vi "SelectionChangedRegEvent.vi"(0 "reference in":refnum<class "DataGridView.lvclass">, 11 "error in (no error)":errorcluster) -> (4 "reference out":refnum<class "DataGridView.lvclass">, 15 "error out":errorcluster)   [LabVIEW 2018, in "DataGridView.lvclass"]
uses:
  DataGridView.lvclass
  System.Windows.Forms
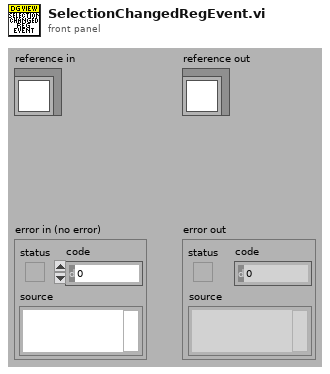
[diagram p1: front panel]
types:
  T1 = typedef "DataGridView.lvclass/ObjectAttributes.ctl" = cluster{"DataGridView":refnum<k24>, "SelectionChangedEvent":refnum<user-event>, "SelectionChanged callback ref":refnum<k27>, "LastSelectedRowIndex":i32, "CellClickEvent":refnum<user-event>, "CellClick callback refnum":refnum<k27>}
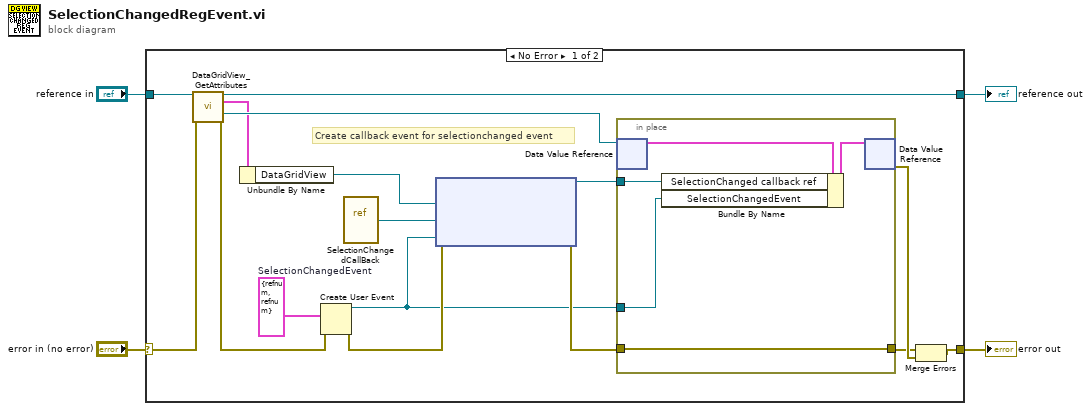
[diagram p0: block diagram]
diagram:
  n1 = case shown="No Error" "error in (no error)" {
    selector: "error in (no error)" -> [w16 w27]
    tunnel: [w14 w27] -> w3
    tunnel: [w18 w26] -> w1
    tunnel: "reference in" -> [w19 w26]
    frame No Error {
      w10 = cluster{"sender":refnum<k24>, "e":refnum<k24>} {"sender"=refnum, "e"=refnum}  # SelectionChangedEvent
      # "Create callback event for selectionchanged event"
      n2 = call "DataGridView_GetAttributes.vi"("reference in"=w19, "error in (no error)"=w16) -> ("reference out"=w18:refnum<class "DataGridView.lvclass">, "Data"=w11:T1, "DataRef"=w17:refnum<data-value>, "error out"=w7:errorcluster)  [unwired: 10 in]
      n3 = Unbundle By Name(w11) -> ("DataGridView"=w9:refnum<k24>)
      n4 = Create User Event(user event datatype=w10, error in=w7) -> (user event=w5:refnum<user-event>, error out=w6:errorcluster)
      n5 = vi-ref "SelectionChangedCallBack.vi"() -> ("vi reference"=w12:refnum<vi>)
      n6 = node(w6, w9, w12, w5) -> (w13:refnum<k27>, w8:errorcluster)  [unwired: 1 in]
      n7 = in-place {
        in-place-border: w8 -> [w24]
        in-place-border: [w24] -> w15
        in-place-border: w13 -> [w22]
        in-place-border: w5 -> [w21]
        n8 = in-place-dvr #1(w17) -> (w23:T1)  [unwired: 1 out]
        n9 = Bundle By Name(cluster=w23, "SelectionChanged callback ref"=w22, "SelectionChangedEvent"=w21) -> (w25:T1)
        n10 = in-place-dvr #1(w25) -> (w20:errorcluster)  [unwired: 1 out]
      }
      n11 = Merge Errors(w15, w20) -> (w14:errorcluster)
    }
    frame Error {
    }
  }
  "error out" <- w3
  "reference out" <- w1
